vi "AI_alarm_to_array.vi"(11 "AI_alarms":T1[](array[typedef])) -> (1 "AI_channel_data":dbl[][](array[numeric]), 2 "TimeStamp":dbl[](array[numeric]), 3 "TimeString":string[](array[string]))   [LabVIEW 2018]
doc: "Timestamp, timestring and corresponding AI_alarm datapoint for each AI_alarm channel."
uses:
  HDF5/AI_alarm_data_cluster.ctl
panel:
  # "Channels in columns\nTimestamp row correpsonds to datapoint in channel data row"
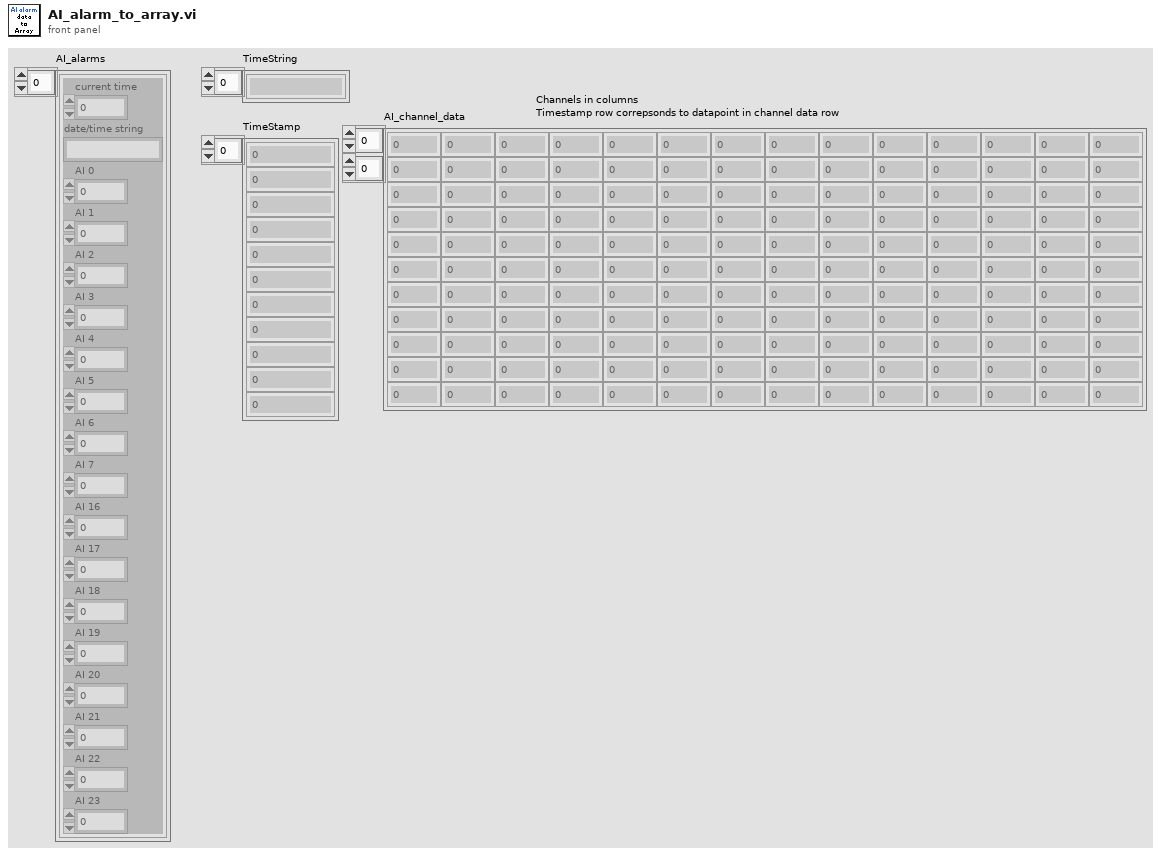
[diagram p1: front panel]
types:
  T1 = typedef "AI_alarm_data_cluster.ctl" = cluster{"current time":dbl, "date/time string":string, "AI 0":dbl, "AI 1":dbl, "AI 2":dbl, "AI 3":dbl, "AI 4":dbl, "AI 5":dbl, "AI 6":dbl, "AI 7":dbl, "AI 16":dbl, "AI 17":dbl, "AI 18":dbl, "AI 19":dbl, "AI 20":dbl, "AI 21":dbl, "AI 22":dbl, "AI 23":dbl}
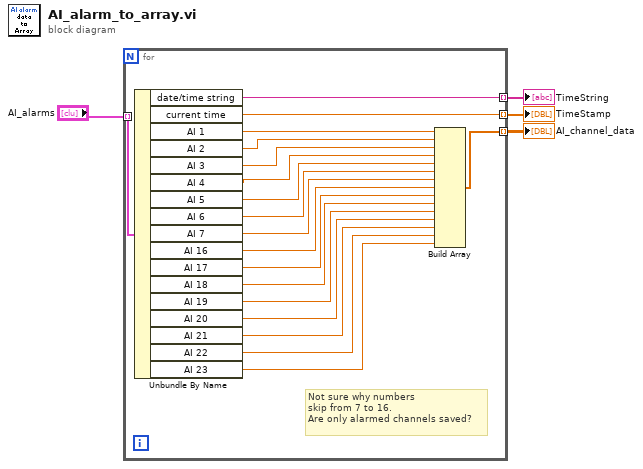
[diagram p0: block diagram]
diagram:
  n1 = for {
    tunnel: "AI_alarms" -> [w23] mode=indexing
    tunnel: [w22] -> w3 mode=indexing
    tunnel: [w21] -> w2 mode=indexing
    tunnel: [w19] -> w4 mode=indexing
    # "Not sure why numbers \nskip from 7 to 16.\nAre only alarmed channels saved?"
    n2 = Unbundle By Name(w23) -> ("date/time string"=w22:string, "current time"=w21:dbl, "AI 1"=w20:dbl, "AI 2"=w18:dbl, "AI 3"=w17:dbl, "AI 4"=w16:dbl, "AI 5"=w15:dbl, "AI 6"=w14:dbl, "AI 7"=w13:dbl, "AI 16"=w12:dbl, "AI 17"=w11:dbl, "AI 18"=w10:dbl, "AI 19"=w9:dbl, "AI 20"=w8:dbl, "AI 21"=w7:dbl, "AI 22"=w6:dbl, "AI 23"=w5:dbl)
    n3 = Build Array(w20, w18, w17, w16, w15, w14, w13, w12, w11, w10, w9, w8, w7, w6, w5) -> (w19:dbl[])
  }
  "AI_channel_data" <- w4
  "TimeString" <- w3
  "TimeStamp" <- w2
